vi "GenerateSignal.vi"(0 "Offset SinZak":dbl, 1 "Offset":dbl, 2 "Frequency":dbl, 3 "Amplitude":dbl, 4 "Phase":dbl, 5 "Radio Buttons 2":T1(radio) caption="Radio Buttons", 6 "stop (F)":bool, 7 "error in (no error)":errorcluster) -> (26 "stopped":bool, 27 "error out":errorcluster)   [LabVIEW 2021]
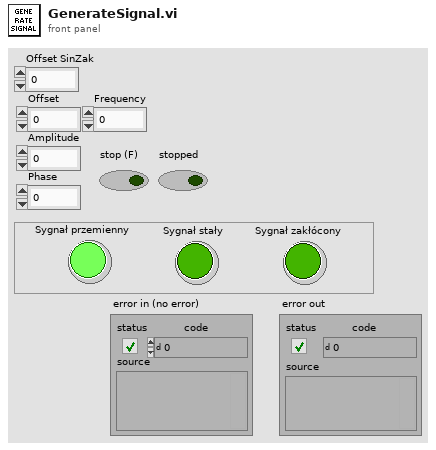
[diagram p1: front panel]
types:
  T1 = enum32{"Sygnał przemienny", "Sygnał stały", "Sygnał zakłócony"}
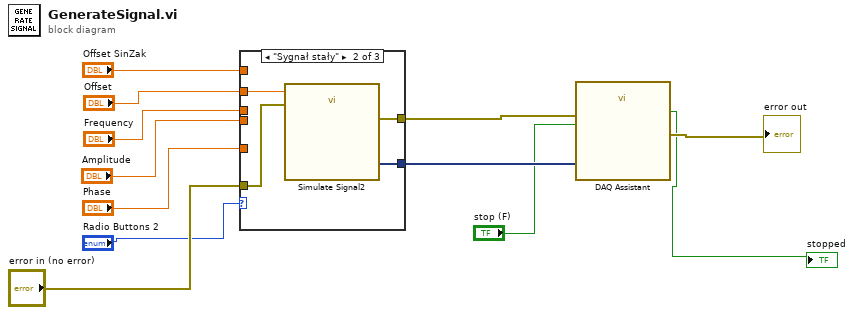
[diagram p0: block diagram]
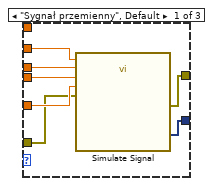
[diagram p2: hidden frame]
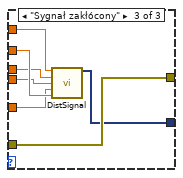
[diagram p3: hidden frame]
diagram:
  n1 = case shown="\"Sygnał stały\"" "Radio Buttons 2" {
    tunnel: "Offset" -> [w19 w23 w29]
    tunnel: "Frequency" -> [w18 _ w28]
    tunnel: "Amplitude" -> [w17 _ w27]
    tunnel: "Phase" -> [w16 _ w26]
    tunnel: "Offset SinZak" -> [_ _ w30]
    tunnel: "error in (no error)" -> [w15 w22 w25]
    tunnel: [w14 w20 w25] -> w4
    tunnel: [w13 w21 w24] -> w3
    frame "Sygnał przemienny", Default {
      n2 = call "Simulate Signal"("Offset"=w19, "Frequency"=w18, "Amplitude"=w17, "Phase"=w16, "error in (no error)"=w15) -> ("Sine"=w13:dynamicdata, "error out"=w14:errorcluster)  [unwired: 9 in]
    }
    frame "Sygnał stały" {
      n3 = call "Simulate Signal2"("Offset"=w23, "error in (no error)"=w22) -> ("DC"=w21:dynamicdata, "error out"=w20:errorcluster)  [unwired: 12 in]
    }
    frame "Sygnał zakłócony" {
      n4 = call "DistSignal.vi"("Offset AC"=w30, "Frequency"=w28, "Amplitude"=w27, "Phase"=w26, "Offset DC"=w29) -> ("Waveform Chart"=w24:dynamicdata)  [unwired: 10 in]
    }
  }
  n5 = call "DAQ Assistant"("data"=w3, "error in"=w4, "stop (F)"="stop (F)") -> ("stopped"=→"stopped":bool, "error out"=→"error out":errorcluster)  [unwired: 14 in, 1 out]
